vi "Test ScollingList.vi"() -> ()   [LabVIEW 2020]
uses:
  Scrolling List Class/Write ListItems.vi
  Scrolling List Class/ScrollingList.lvclass
panel:
  out "List Picture":picture
  out "Selection":string
  out "Background Picture":picture
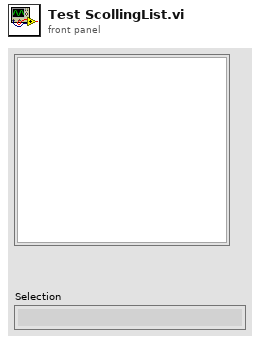
[diagram p1: front panel]
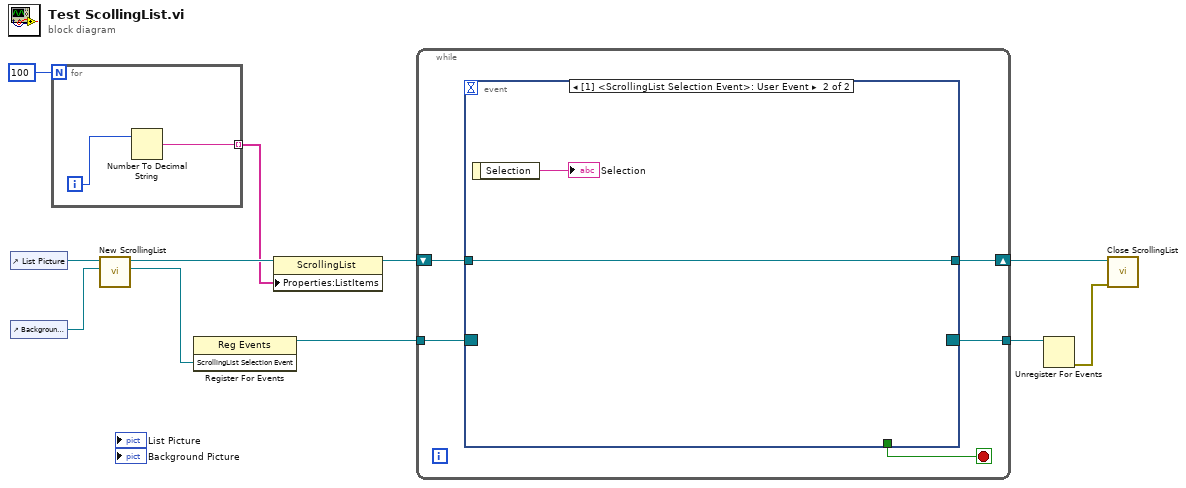
[diagram p0: block diagram]
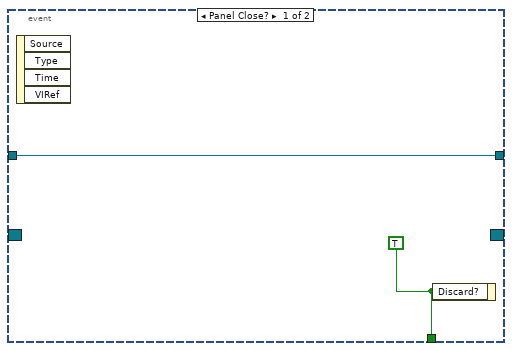
[diagram p2: hidden frame]
diagram:
  n1 = control-ref of="List Picture"() -> (w10:refnum<vi>)
  n2 = control-ref of="Background Picture"() -> (w9:refnum<vi>)
  n3 = for {
    N: 100 -> [_]
    tunnel: [w12] -> w1 mode=indexing
    i -> [w13]
    n4 = Number To Decimal String(number=w13) -> (decimal integer string=w12:string)  [unwired: 1 in]
  }
  n5 = call "New ScrollingList.vi"("BackgroundPicture Ref"=w9, "Reference"=w10) -> ("ScrollingList Selection Event"=w8:refnum<user-event>, "ScrollingList out"=w11:refnum<class "ScrollingList.lvclass">)  [unwired: 7 in, 1 out]
  n6 = register-events(w8) -> (reference out=w6:refnum<event-registration>)  [unwired: 2 in, 1 out]
  n7 = property class="ScrollingList"(reference=w11, "Properties:ListItems"=w1) -> (reference out=w3:refnum<class "ScrollingList.lvclass">)  [unwired: 1 in, 1 out]
  n8 = while {
    shift-right: [w17] -> w7
    shift-left: w3 -> [w16]
    tunnel: w6 -> [w15]
    tunnel: [w14] -> w5
    stop <- w18 stop-if-true
    n9 = event shown="[1] <ScrollingList Selection Event>: User Event" {
      selector: w15 -> [_ _]
      dyn-events: [_ _] -> w14
      timeout: _ -> [_ _]
      tunnel: [w20 _] -> w18
      tunnel: [w19 w21] -> w17
      tunnel: w16 -> [w19 w21]
      event Panel Close? {
        w20 = TRUE ("Discard?")
        n10 = event-data() -> ()  [unwired: 1 in, 4 out]
        n11 = event-data("Discard?"=w20) -> ()  [unwired: 1 in, 1 out]
      }
      event User Event {
        n12 = event-data() -> ("Selection"=→"Selection":string)  [unwired: 1 in]
      }
    }
  }
  n13 = Unregister For Events(event registration refnum=w5) -> (error out=w4:errorcluster)  [unwired: 1 in]
  n14 = call "Close ScrollingList.vi"("error in (no error)"=w4, "ScrollingList in"=w7) -> ()  [unwired: 9 in, 1 out]
